vi "CleanErr56-66.vi"(8 "error in (no error)":errorcluster) -> (0 "error out":errorcluster, 3 "Errors":T1)   [LabVIEW 2020]
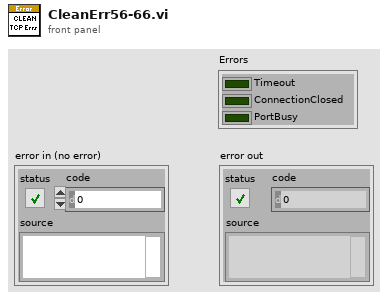
[diagram p1: front panel]
types:
  T1 = cluster{"Timeout":bool, "ConnectionClosed":bool, "PortBusy":bool}
  T2 = cluster{"Boolean array[0]":bool, "Boolean array[1]":bool, "Boolean array[2]":bool}
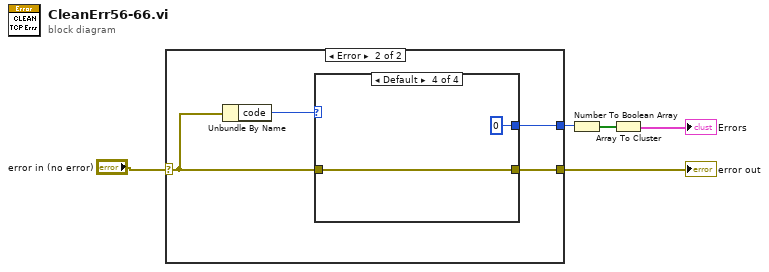
[diagram p0: block diagram]
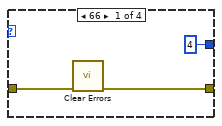
[diagram p3: hidden frame]
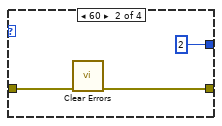
[diagram p4: hidden frame]
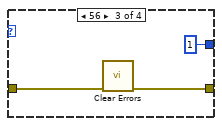
[diagram p5: hidden frame]
diagram:
  n1 = case shown="Error" "error in (no error)" {
    selector: "error in (no error)" -> [w6 w9]
    tunnel: [w6 w8] -> w4
    tunnel: [_ w7] -> w1
    frame No Error {
    }
    frame Error {
      n2 = Unbundle By Name(w9) -> ("code"=w10:i32)
      n3 = case shown="Default" w10 {
        tunnel: w9 -> [w13 w16 w18 w21]
        tunnel: [w12 w15 w19 w21] -> w8
        tunnel: [4 2 1 0] -> w7
        frame 66 {
          n4 = call <vilib>:"Clear Errors.vi"("error in (no error)"=w13) -> ("error out"=w12:errorcluster)  [unwired: 5 in, 1 out]
        }
        frame 60 {
          n5 = call <vilib>:"Clear Errors.vi"("error in (no error)"=w16) -> ("error out"=w15:errorcluster)  [unwired: 5 in, 1 out]
        }
        frame 56 {
          n6 = call <vilib>:"Clear Errors.vi"("error in (no error)"=w18) -> ("error out"=w19:errorcluster)  [unwired: 5 in, 1 out]
        }
        frame Default {
        }
      }
    }
  }
  "error out" <- w4
  n7 = Number To Boolean Array(number=w1) -> (Boolean array=w3:bool[])
  n8 = Array To Cluster(array=w3) -> (cluster=→"Errors":T2)
